vi "Deinit.vi"(8 "error in (no error)":errorcluster, 11 "EEH - User Event in":refnum<class "EngineEventHandler-UserEvent.lvclass">) -> (0 "error out":errorcluster)   [LabVIEW 2020, in "GLF.lvlib" / "EngineEventHandler-UserEvent.lvclass"]
uses:
  EngineEventHandler-UserEvent.lvclass
  EngineEventHandler-UserEvent.lvclass/EngineEventHandler-UserEvent.ctl
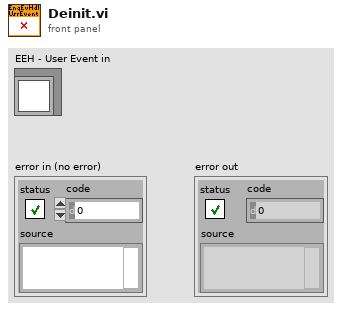
[diagram p1: front panel]
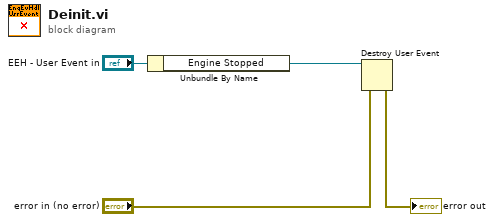
[diagram p0: block diagram]
diagram:
  n1 = Unbundle By Name("EEH - User Event in") -> ("Engine Stopped"=w2:refnum<user-event>)
  n2 = Destroy User Event(user event=w2, error in="error in (no error)") -> (error out=→"error out":errorcluster)
